vi "Initialize DAQ.vi"(8 "error in (no error)":errorcluster, 10 "DAQ Settings":T2, 11 "DAQmx Resource":tag) -> (0 "error out":errorcluster, 3 "DAQmx Tasks":T1)   [LabVIEW 2025]
uses:
  <vilib>/DAQmx/write.llb/DAQmx Write (Digital Wfm 1Chan NSamp).vi
  <vilib>/DAQmx/create/channels.llb/DAQmx Create Channel (CO-Pulse Generation-Frequency).vi
  <vilib>/DAQmx/configure/timing.llb/DAQmx Timing (Implicit).vi
  <vilib>/Waveform/DWDTOps.llb/DWDT Append Digital Samples.vi
  <vilib>/Waveform/DWDTOps.llb/DWDT Digital Size.vi
  <vilib>/DAQmx/configure/timing.llb/DAQmx Timing (Sample Clock).vi
  <vilib>/Waveform/DWDTOps.llb/DWDT Uncompress Digital.vi
  <vilib>/DAQmx/miscellaneous.llb/DAQmx Fill In Error Info.vi
  <resource>/objmgr/daqmx.rc
panel:
  out "Actual Sample Rate Frequency":dbl
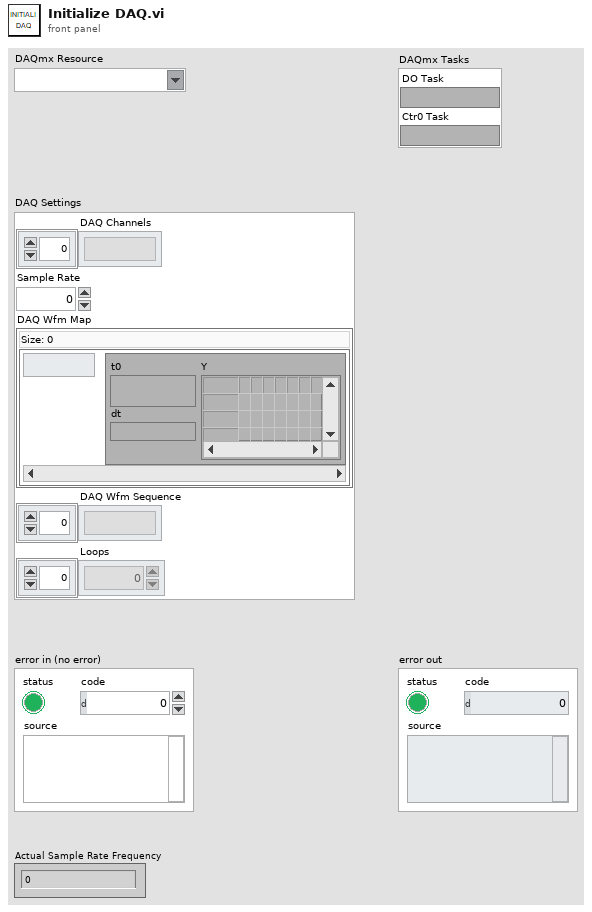
[diagram p1: front panel]
types:
  T1 = cluster{"DO Task":refnum<k21>, "Ctr0 Task":refnum<k21>}
  T2 = cluster{"DAQ Channels":string[], "Sample Rate":dbl, "DAQ Wfm Map":map{string, digitalwaveform}, "DAQ Wfm Sequence":string[], "Loops":i32[]}
  T3 = cluster{"task out":refnum<k21>, "task out":refnum<k21>}
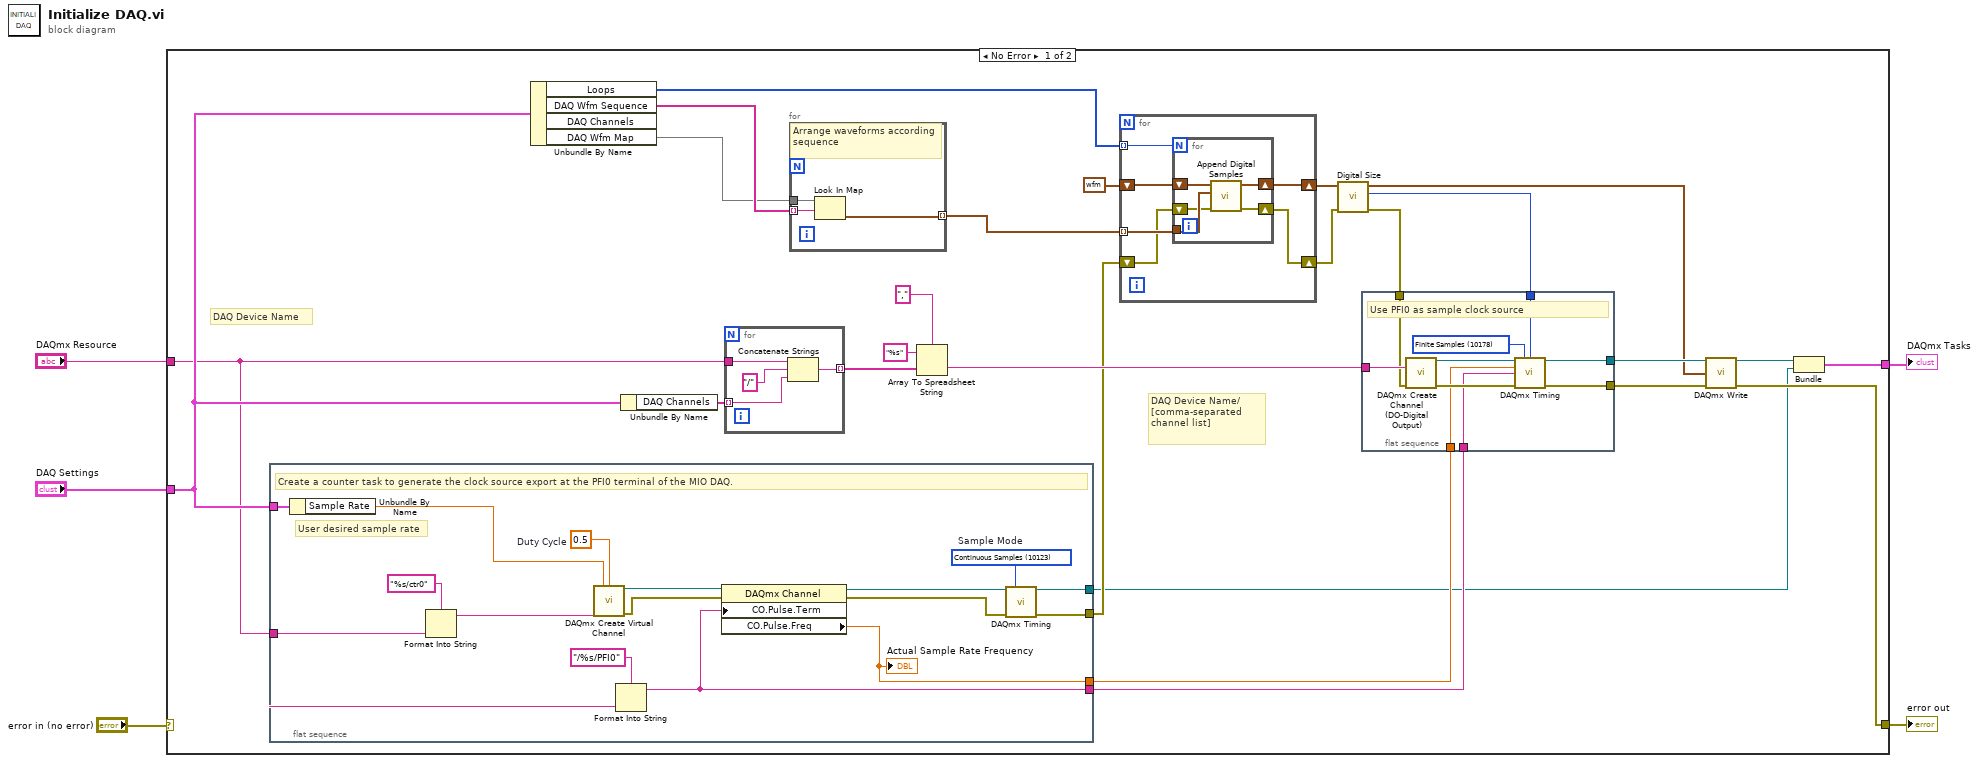
[diagram p0: block diagram]
diagram:
  n1 = case shown="No Error" "error in (no error)" {
    selector: "error in (no error)" -> [_ w76]
    tunnel: [w21 w76] -> w5
    tunnel: "DAQmx Resource" -> [w19 _]
    tunnel: "DAQ Settings" -> [w30 _]
    tunnel: [w10 _] -> w1
    frame No Error {
      # "DAQ Device Name/[comma-separated channel list]"
      # "DAQ Device Name"
      n2 = flat-sequence {
        tunnel: w30 -> [w57]
        tunnel: w19 -> [w46]
        tunnel: [w45] -> w18
        tunnel: [w44] -> w13
        tunnel: [w43] -> w17
        tunnel: [w42] -> w9
        frame #0 {
          w51 = 0.5  # Duty Cycle
          w56 = 10123 items=["Finite Samples"=10178, "Continuous Samples"=10123, "Hardware Timed Single Point"=12522]  # Sample Mode
          # "User desired sample rate"
          # "Create a counter task to generate the clock source export at the PFI0 terminal of the MIO DAQ."
          n3 = Unbundle By Name(w57) -> ("Sample Rate"=w50:dbl)
          n4 = Format Into String(format string="%s/ctr0", w46) -> (resulting string=w48:string)  [unwired: 2 in, 1 out]
          n5 = call-poly <vilib>:"DAQmx Create Virtual Channel.vi"("frequency"=w50, "duty cycle"=w51, "counter"=w48) -> ("task out"=w55:refnum<k21>, "error out"=w54:errorcluster)  [unwired: 11 in]
          n6 = Format Into String(format string="/%s/PFI0", w46) -> (resulting string=w43:string)  [unwired: 2 in, 1 out]
          n7 = property class="DAQmx Channel"(reference=w55, error in=w54, "CO.Pulse.Term"=w43) -> (reference out=w52:refnum<k21>, error out=w53:errorcluster, "CO.Pulse.Freq"=w45:dbl)
          "Actual Sample Rate Frequency" <- w45
          n8 = call-poly <vilib>:"DAQmx Timing.vi"("task/channels in"=w52, "sample mode"=w56, "error in"=w53) -> ("task out"=w42:refnum<k21>, "error out"=w44:errorcluster)  [unwired: 11 in]
        }
      }
      n9 = Unbundle By Name(w30) -> ("Loops"=w7:i32[], "DAQ Wfm Sequence"=w31:string[], "DAQ Wfm Map"=w24:map{string, digitalwaveform})  [unwired: 1 out]
      n10 = Unbundle By Name(w30) -> ("DAQ Channels"=w29:string[])
      n11 = for {
        tunnel: w19 -> [w75]
        tunnel: w29 -> [w73] mode=indexing
        tunnel: [w72] -> w28 mode=indexing
        n12 = Concatenate Strings(w75, "/", w73) -> (w72:string)
      }
      n13 = for {
        tunnel: w31 -> [w71] mode=indexing
        tunnel: w24 -> [w70]
        tunnel: [w69] -> w23 mode=indexing
        # "Arrange waveforms according sequence"
        n14 = Look In Map(map=w70, key=w71) -> (value=w69:digitalwaveform)  [unwired: 1 in, 1 out]
      }
      n15 = Array To Spreadsheet String(delimiter (Tab)=",", array=w28, 3:"%s" ("format string")) -> (spreadsheet string=w25:string)
      n16 = for {
        shift-right: [w62] -> w16
        shift-left: digitalwaveform {"t0"=timestamp(0 s since 1904-01-01), "dt"=0.0, "Y"={"transitions"=[], "data"=[]}} ("digital waveform out") -> [w63]
        tunnel: w23 -> [w61] mode=indexing
        shift-right: [w59] -> w14
        shift-left: w13 -> [w60]
        tunnel: w7 -> [w58] mode=indexing
        n17 = for {
          N: w58 -> [_]
          tunnel: w61 -> [w66]
          shift-right: [w67] -> w62
          shift-left: w63 -> [w68]
          shift-right: [w64] -> w59
          shift-left: w60 -> [w65]
          n18 = call-poly <vilib>:"Append Digital Samples.vi"("error in (no error)"=w65, "digital waveform B"=w66, "digital waveform A"=w68) -> ("error out"=w64:errorcluster, "digital waveform out"=w67:digitalwaveform)  [unwired: 7 in]
        }
      }
      n19 = call-poly <vilib>:"Digital Size.vi"("error in (no error)"=w14, "digital waveform in"=w16) -> ("error out"=w12:errorcluster, "number of samples"=w15:i32, "digital waveform out"=w8:digitalwaveform)  [unwired: 6 in, 1 out]
      n20 = flat-sequence {
        tunnel: w25 -> [w41]
        tunnel: [w37] -> w20
        tunnel: w18 -> [w36]
        tunnel: w17 -> [w35]
        tunnel: w15 -> [w34]
        tunnel: w12 -> [w33]
        tunnel: [w32] -> w11
        frame #0 {
          w38 = 10178 items=["Finite Samples"=10178, "Continuous Samples"=10123, "Hardware Timed Single Point"=12522] ("sample mode")
          # "Use PFI0 as sample clock source"
          n21 = call <vilib>:"DAQmx Create Channel (DO-Digital Output).vi"("lines"=w41, "error in"=w33) -> ("task out"=w39:refnum<k21>, "error out"=w40:errorcluster)  [unwired: 12 in]
          n22 = call-poly <vilib>:"DAQmx Timing.vi"("task/channels in"=w39, "sample mode"=w38, "samples per channel"=w34, "rate"=w36, "source"=w35, "error in"=w40) -> ("task out"=w37:refnum<k21>, "error out"=w32:errorcluster)  [unwired: 8 in]
        }
      }
      n23 = call-poly <vilib>:"DAQmx Write.vi"("task/channels in"=w20, "data"=w8, "error in"=w11) -> ("task out"=w22:refnum<k21>, "error out"=w21:errorcluster)  [unwired: 10 in, 1 out]
      n24 = Bundle("task out"=w22, "task out"=w9) -> (w10:T3)  [unwired: 1 in]
    }
    frame Error {
    }
  }
  "error out" <- w5
  "DAQmx Tasks" <- w1
